vi "Refresh Tag Exchange Prefix and Suffix.vi"(6 "Tag Exchange Tab References":T1, 8 "error in (no error)":errorcluster, 11 "E2E editor node in":refnum<data-value>) -> (0 "error out":errorcluster, 3 "E2E editor node out":refnum<data-value>)   [LabVIEW 2015, in "E2E Tag Exchange editor node.lvclass"]
uses:
  E2E Tag Exchange editor node.lvclass
  Tag Exchange Tab References.ctl
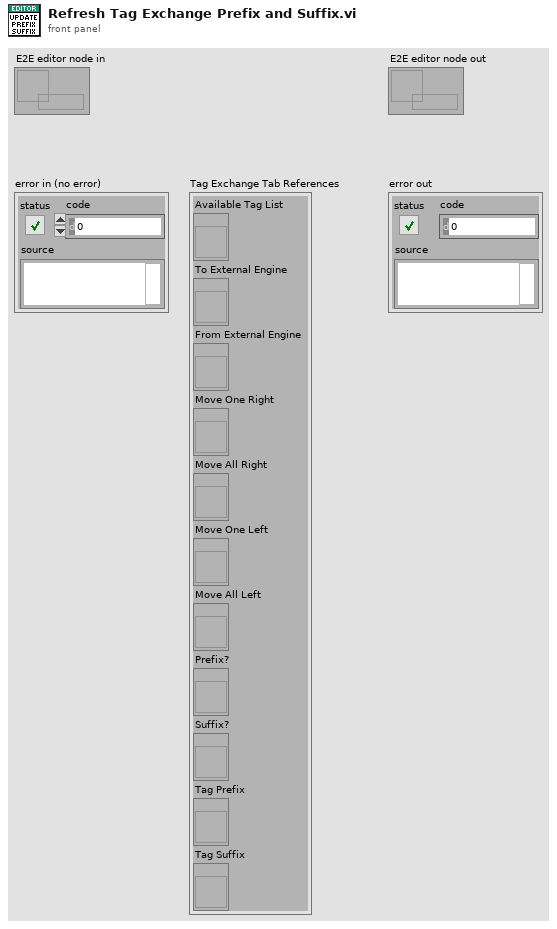
[diagram p1: front panel]
types:
  T1 = typedef "E2E Tag Exchange editor node.lvclass/Tag Exchange Tab References.ctl" = cluster{"Available Tag List":refnum<vi>, "To External Engine":refnum<vi>, "From External Engine":refnum<vi>, "Move One Right":refnum<vi>, "Move All Right":refnum<vi>, "Move One Left":refnum<vi>, "Move All Left":refnum<vi>, "Prefix?":refnum<vi>, "Suffix?":refnum<vi>, "Tag Prefix":refnum<vi>, "Tag Suffix":refnum<vi>}
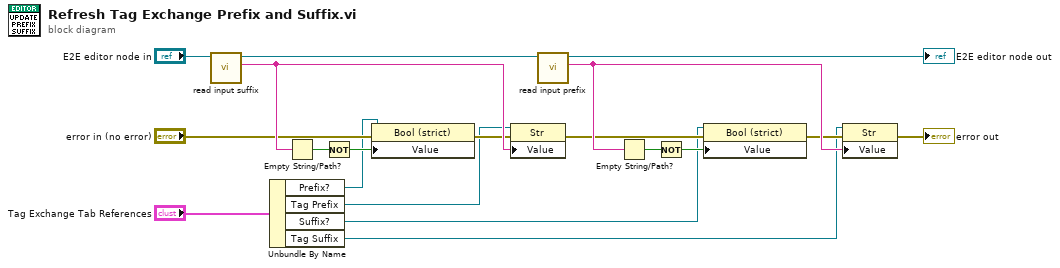
[diagram p0: block diagram]
diagram:
  n1 = call "read input suffix.vi"("E2E editor node in"="E2E editor node in") -> ("Input Suffix"=w13:string, "E2E editor node out"=w9:refnum<data-value>)  [unwired: 8 in, 1 out]
  n2 = Unbundle By Name("Tag Exchange Tab References") -> ("Prefix?"=w5:refnum<vi>, "Tag Prefix"=w4:refnum<vi>, "Suffix?"=w3:refnum<vi>, "Tag Suffix"=w2:refnum<vi>)
  n3 = Empty String/Path?(string/path=w13) -> (empty?=w10:bool)
  n4 = Not(x=w10) -> (.not. x?=w11:bool)
  n5 = property class="Bool (strict)"(reference=w5, error in="error in (no error)", "Value"=w11) -> (error out=w12:errorcluster)  [unwired: 1 out]
  n6 = property class="Str"(reference=w4, error in=w12, "Value"=w13) -> (error out=w17:errorcluster)  [unwired: 1 out]
  n7 = call "read input prefix.vi"("E2E editor node in"=w9) -> ("Input Prefix"=w18:string, "E2E editor node out"=→"E2E editor node out":refnum<data-value>)  [unwired: 8 in, 1 out]
  n8 = Empty String/Path?(string/path=w18) -> (empty?=w16:bool)
  n9 = Not(x=w16) -> (.not. x?=w15:bool)
  n10 = property class="Bool (strict)"(reference=w3, error in=w17, "Value"=w15) -> (error out=w14:errorcluster)  [unwired: 1 out]
  n11 = property class="Str"(reference=w2, error in=w14, "Value"=w18) -> (error out=→"error out":errorcluster)  [unwired: 1 out]
